vi "DpcCloseData.vi"(8 "Error In":errorcluster, 11 "Device Handle":u32) -> (0 "Error Out":errorcluster, 3 "Device Handle":u32)   [LabVIEW 2011, in "LVH-Adept.lvlib" / "DPCUTIL.lvlib"]
uses:
  DPCUTIL.lvlib
  Private/Type Defs/Error.ctl
  Resources/dpcutil.dll
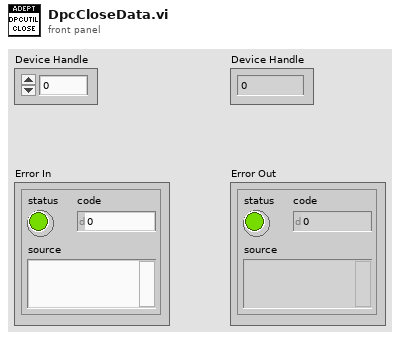
[diagram p1: front panel]
types:
  T1 = typedef "LVH-Adept.lvlib/DPCUTIL.lvlib/Error.ctl" = enum16{"Unknown", "Open Data", "Wait For Transaction", "Put Reg", "Get Reg", "Close Data"}
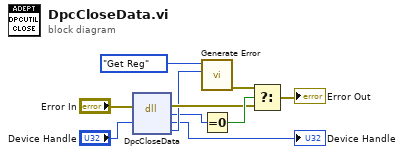
[diagram p0: block diagram]
diagram:
  n1 = dll-call lib="C:/github/labviewhacker/LVH-Adept/LabVIEW/vi.lib/LabVIEW Hacker/Adept/Private/Resources/dpcutil.*" fn="DpcCloseData"(error in="Error In", "hif"="Device Handle") -> (error out=w5:errorcluster, w2:i32, "hif"=→"Device Handle":u32, "perc"=w3:i32)  [unwired: 3 in, 1 out]
  n2 = call "Generate Error.vi"("Adept Error Code"=w3, "DPCUTIL Error"=Error."Get Reg") -> ("Error Out"=w10:errorcluster)  [unwired: 9 in]
  n3 = Equal To 0?(x=w2) -> (x = 0?=w9:bool)
  n4 = Select(t=w10, s=w9, f=w5) -> (s? t:f=→"Error Out":errorcluster)
